vi "Cluster To String.vi"(8 "error in (no error)":errorcluster caption="错误输入（无错误）", 11 "face Parameter":T1) -> (0 "error out":errorcluster, 3 "String":string)   [LabVIEW 2025]
uses:
  <vilib>/Utility/Data Type/NI_Data Type.lvlib
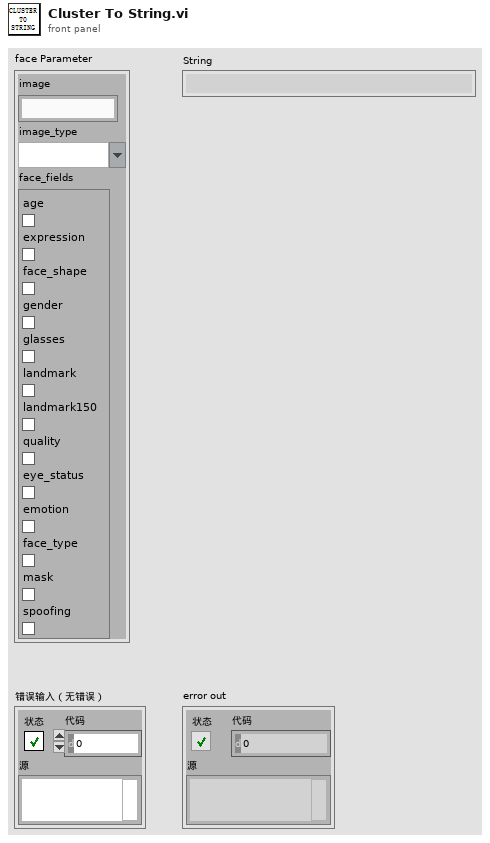
[diagram p1: front panel]
types:
  T1 = cluster{"image":string, "image_type":string, "face_fields ":cluster{"age":bool, "expression":bool, "face_shape":bool, "gender":bool, "glasses":bool, "landmark":bool, "landmark150":bool, "quality":bool, "eye_status":bool, "emotion":bool, "face_type":bool, "mask":bool, "spoofing":bool}}
  T2 = cluster{"age":bool, "expression":bool, "face_shape":bool, "gender":bool, "glasses":bool, "landmark":bool, "landmark150":bool, "quality":bool, "eye_status":bool, "emotion":bool, "face_type":bool, "mask":bool, "spoofing":bool}
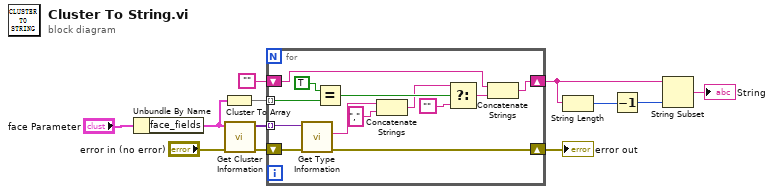
[diagram p0: block diagram]
diagram:
  n1 = Unbundle By Name("face Parameter") -> ("face_fields"=w10:T2)
  n2 = Cluster To Array(cluster=w10) -> (array=w11:bool[])
  n3 = call <vilib>:"Get Cluster Information.vi"("error in (no error)"="error in (no error)", "variant"=w10) -> ("error out"=w3:errorcluster, "cluster elements"=w9:variant[])  [unwired: 8 in]
  n4 = for {
    tunnel: w11 -> [w25] mode=indexing
    tunnel: w9 -> [w23] mode=indexing
    shift-right: [w17] -> w7
    shift-left: "" -> [w22]
    shift-right: [w13] -> w1
    shift-left: w3 -> [w14]
    n5 = call <vilib>:"Get Type Information.vi"("error in (no error)"=w14, "variant"=w23) -> ("error out"=w13:errorcluster, "name"=w21:string)  [unwired: 5 in, 3 out]
    n6 = Equal?(x=TRUE, y=w25) -> (x = y?=w20:bool)
    n7 = Concatenate Strings(w21, "," ("字符串")) -> (w15:string)
    n8 = Select(t=w15, s=w20, f="") -> (s? t:f=w18:string)
    n9 = Concatenate Strings(w22, w18) -> (w17:string)
  }
  "error out" <- w1
  n10 = String Length(string=w7) -> (length=w6:i32)
  n11 = Decrement(x=w6) -> (x-1=w5:i32)
  n12 = String Subset(string=w7, length (rest)=w5) -> (substring=→"String":string)  [unwired: 1 in]
